vi "CAN Jaguar Get Output.vi"(8 "error in (no error)":errorcluster, 11 "CAN Jaguar Ref":T1={"Device Number"=0, "Control Mode"=enum."Percent VBus", "Inverted"=FALSE, "Semaphore"=refnum, "Max Vout"=12.0, "DevStatus"={"status"=FALSE, "code"=0, "source"=""}}) -> (0 "error out":errorcluster, 2 "Output Set Point":dbl, 3 "CAN Jaguar Ref Out":T1={"Device Number"=0, "Control Mode"=enum."Percent VBus", "Inverted"=FALSE, "Semaphore"=refnum, "Max Vout"=12.0, "DevStatus"={"status"=FALSE, "code"=0, "source"=""}})   [LabVIEW 2009, in "CAN.lvlib"]
uses:
  CAN.lvlib
  SubVIs/CAN Jaguar Ref.ctl
  SubVIs/CAN Jaguar Control Mode.ctl
  SubVIs/CAN Motor Message IDs.ctl
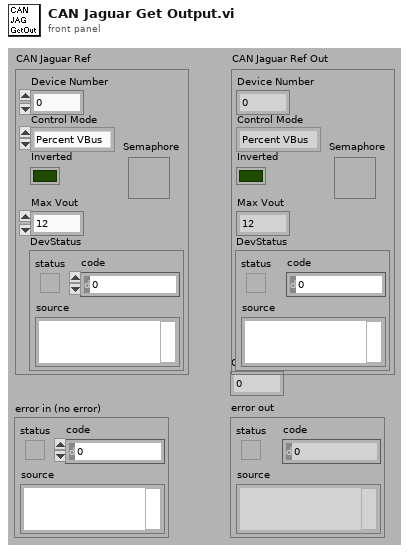
[diagram p1: front panel]
types:
  T1 = typedef "CAN.lvlib/CAN Jaguar Ref.ctl" = cluster{"Device Number":u8, "Control Mode":T2, "Inverted":bool, "Semaphore":T3, "Max Vout":dbl, "DevStatus":errorcluster}
  T2 = typedef "CAN.lvlib/CAN Jaguar Control Mode.ctl" = enum16{"Percent VBus", "Speed", "Position", "Current"}
  T3 = typedef "Semaphore RefNum" = refnum<k1>
  T4 = enum16{"big-endian, network order", "native, host order", "little-endian"}
  T5 = typedef "CAN.lvlib/CAN Motor Message IDs.ctl" = u32
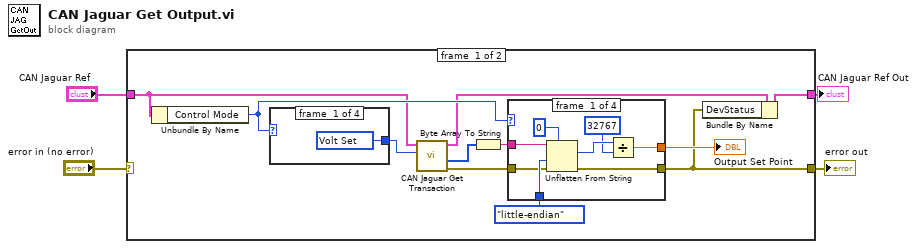
[diagram p0: block diagram]
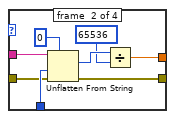
[diagram p2: hidden frame]
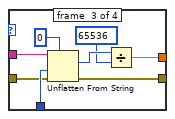
[diagram p3: hidden frame]
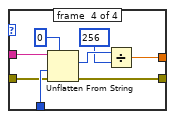
[diagram p4: hidden frame]
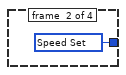
[diagram p5: hidden frame]
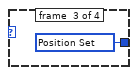
[diagram p6: hidden frame]
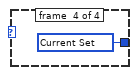
[diagram p7: hidden frame]
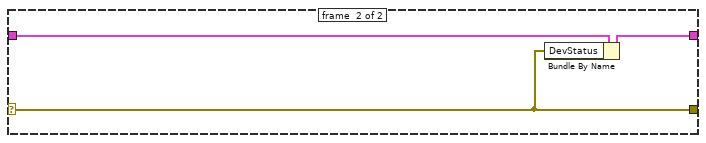
[diagram p8: hidden frame]
diagram:
  n1 = case shown="No Error" "error in (no error)" {
    selector: "error in (no error)" -> [_ w52]
    tunnel: [w15 w53] -> w4
    tunnel: "CAN Jaguar Ref" -> [w9 w54]
    tunnel: [w11 w52] -> w2
    frame #0 {
      n2 = Unbundle By Name(w9) -> ("Control Mode"=w10:T2)
      n3 = case shown="\"Percent VBus\"" w10 {
        tunnel: [w48 w49 w50 w51] -> w5
        frame #0 {
          w48 = T5 33685632 items=["Volt Enable"=33685504, "Volt Disable"=33685568, "Volt Set"=33685632, "Volt Set Ramp"=33685696, "Speed Enable"=33686528, "Speed Disable"=33686592, "Speed Set"=33686656, "Speed P"=33686720, "Speed I"=33686784, "Speed D"=33686848, "Speed Ref"=33686912, "Position Enable"=33688576, "Position Disable"=33688640, "Position Set"=33688704, "Position P"=33688768, "Position I"=33688832, "Position D"=33688896, "Position Ref"=33688960, "Current Enable"=33689600, "Current Disable"=33689664, "Current Set"=33689728, "Current P"=33689792, "Current I"=33689856, "Current D"=33689920, "Status VOut"=33690624, "Status VBus"=33690688, "Status Current"=33690752, "Status Temp"=33690816, "Status Position"=33690880, "Status Speed"=33690944, "Status Limit"=33691008, "Status Fault"=33691072, "Status Power"=33691136, "Config Num Brushes"=33692672, "Config Encoder Lines"=33692736, "Config Pot Turns"=33692800, "Config Brake Coast"=33692864, "Config Limit Mode"=33692928, "Config Limit Fwd"=33692992, "Config Limit Rev"=33693056, "Config Max VOut"=33693120, "Config Fault Time"=33693184, "Motor Ack"=33693696] ("CAN Motor Message IDs")
        }
        frame #1 {
          w49 = T5 33686656 items=["Volt Enable"=33685504, "Volt Disable"=33685568, "Volt Set"=33685632, "Volt Set Ramp"=33685696, "Speed Enable"=33686528, "Speed Disable"=33686592, "Speed Set"=33686656, "Speed P"=33686720, "Speed I"=33686784, "Speed D"=33686848, "Speed Ref"=33686912, "Position Enable"=33688576, "Position Disable"=33688640, "Position Set"=33688704, "Position P"=33688768, "Position I"=33688832, "Position D"=33688896, "Position Ref"=33688960, "Current Enable"=33689600, "Current Disable"=33689664, "Current Set"=33689728, "Current P"=33689792, "Current I"=33689856, "Current D"=33689920, "Status VOut"=33690624, "Status VBus"=33690688, "Status Current"=33690752, "Status Temp"=33690816, "Status Position"=33690880, "Status Speed"=33690944, "Status Limit"=33691008, "Status Fault"=33691072, "Status Power"=33691136, "Config Num Brushes"=33692672, "Config Encoder Lines"=33692736, "Config Pot Turns"=33692800, "Config Brake Coast"=33692864, "Config Limit Mode"=33692928, "Config Limit Fwd"=33692992, "Config Limit Rev"=33693056, "Config Max VOut"=33693120, "Config Fault Time"=33693184, "Motor Ack"=33693696] ("CAN Motor Message IDs")
        }
        frame #2 {
          w50 = T5 33688704 items=["Volt Enable"=33685504, "Volt Disable"=33685568, "Volt Set"=33685632, "Volt Set Ramp"=33685696, "Speed Enable"=33686528, "Speed Disable"=33686592, "Speed Set"=33686656, "Speed P"=33686720, "Speed I"=33686784, "Speed D"=33686848, "Speed Ref"=33686912, "Position Enable"=33688576, "Position Disable"=33688640, "Position Set"=33688704, "Position P"=33688768, "Position I"=33688832, "Position D"=33688896, "Position Ref"=33688960, "Current Enable"=33689600, "Current Disable"=33689664, "Current Set"=33689728, "Current P"=33689792, "Current I"=33689856, "Current D"=33689920, "Status VOut"=33690624, "Status VBus"=33690688, "Status Current"=33690752, "Status Temp"=33690816, "Status Position"=33690880, "Status Speed"=33690944, "Status Limit"=33691008, "Status Fault"=33691072, "Status Power"=33691136, "Config Num Brushes"=33692672, "Config Encoder Lines"=33692736, "Config Pot Turns"=33692800, "Config Brake Coast"=33692864, "Config Limit Mode"=33692928, "Config Limit Fwd"=33692992, "Config Limit Rev"=33693056, "Config Max VOut"=33693120, "Config Fault Time"=33693184, "Motor Ack"=33693696] ("CAN Motor Message IDs")
        }
        frame #3 {
          w51 = T5 33689728 items=["Volt Enable"=33685504, "Volt Disable"=33685568, "Volt Set"=33685632, "Volt Set Ramp"=33685696, "Speed Enable"=33686528, "Speed Disable"=33686592, "Speed Set"=33686656, "Speed P"=33686720, "Speed I"=33686784, "Speed D"=33686848, "Speed Ref"=33686912, "Position Enable"=33688576, "Position Disable"=33688640, "Position Set"=33688704, "Position P"=33688768, "Position I"=33688832, "Position D"=33688896, "Position Ref"=33688960, "Current Enable"=33689600, "Current Disable"=33689664, "Current Set"=33689728, "Current P"=33689792, "Current I"=33689856, "Current D"=33689920, "Status VOut"=33690624, "Status VBus"=33690688, "Status Current"=33690752, "Status Temp"=33690816, "Status Position"=33690880, "Status Speed"=33690944, "Status Limit"=33691008, "Status Fault"=33691072, "Status Power"=33691136, "Config Num Brushes"=33692672, "Config Encoder Lines"=33692736, "Config Pot Turns"=33692800, "Config Brake Coast"=33692864, "Config Limit Mode"=33692928, "Config Limit Fwd"=33692992, "Config Limit Rev"=33693056, "Config Max VOut"=33693120, "Config Fault Time"=33693184, "Motor Ack"=33693696] ("CAN Motor Message IDs")
        }
      }
      n4 = call "CAN Jaguar Get Transaction.vi"("Message ID"=w5, "CAN Jaguar Ref"=w9) -> ("error out"=w6:errorcluster, "Data"=w7:u8[], "CAN Jaguar Ref Out"=w8:T1)  [unwired: 1 in, 6 out]
      n5 = Byte Array To String(unsigned byte array=w7) -> (string=w12:string)
      n6 = case shown="\"Current\"" w10 {
        tunnel: [w17 w25 w33 w42] -> w14
        tunnel: T4."little-endian" ("byte order (0:big-endian, network order)") -> [w22 w31 w39 w47]
        tunnel: w12 -> [w20 w29 w37 w45]
        tunnel: w6 -> [w19 w28 w36 w44]
        tunnel: [w18 w27 w35 w43] -> w11
        frame #0 {
          n7 = Unflatten From String(type=i16 0 ("Voltage"), binary string=w20, byte order (0:big-endian, network order)=w22, error in (no error)=w19) -> (value=w23:i16, error out=w18:errorcluster)  [unwired: 2 out]
          n8 = Divide(x=w23, y=i16 32767) -> (x/y=w17:dbl)
        }
        frame #1 {
          n9 = Unflatten From String(type=0 ("Voltage"), binary string=w29, byte order (0:big-endian, network order)=w31, error in (no error)=w28) -> (value=w26:i32, error out=w27:errorcluster)  [unwired: 2 out]
          n10 = Divide(x=w26, y=65536 ("x")) -> (x/y=w25:dbl)
        }
        frame #2 {
          n11 = Unflatten From String(type=0 ("Voltage"), binary string=w37, byte order (0:big-endian, network order)=w39, error in (no error)=w36) -> (value=w34:i32, error out=w35:errorcluster)  [unwired: 2 out]
          n12 = Divide(x=w34, y=65536 ("x")) -> (x/y=w33:dbl)
        }
        frame #3 {
          n13 = Unflatten From String(type=i16 0 ("Voltage"), binary string=w45, byte order (0:big-endian, network order)=w47, error in (no error)=w44) -> (value=w41:i16, error out=w43:errorcluster)  [unwired: 2 out]
          n14 = Divide(x=w41, y=i16 256) -> (x/y=w42:dbl)
        }
      }
      "Output Set Point" <- w14
      n15 = Bundle By Name(cluster=w8, "DevStatus"=w11) -> (w15:T1)
    }
    frame #1 {
      n16 = Bundle By Name(cluster=w54, "DevStatus"=w52) -> (w53:T1)
    }
  }
  "CAN Jaguar Ref Out" <- w4
  "error out" <- w2
